vi "WLC for FA-50%GC_YCC.vi"() -> ()   [LabVIEW 2014]
uses:
  <vilib>/Utility/file.llb/Read From Spreadsheet File (DBL).vi
  <vilib>/gmath/NumericalOptimization/Nonlinear Curve Fit LM formula string.vi
  <vilib>/Utility/file.llb/Write To Spreadsheet File (DBL).vi
  <vilib>/gmath/NI_Gmath.lvlib
panel:
  out "reduced dsDNA (bp)":dbl=1002.0
  out "ssDNA generated (nt)":dbl
  out "Force Array  for activated best fit (pN)":dbl[](array[numeric])
  out "Extension array for activated best fit (nm)":dbl[](array[numeric])
  out "Force Array  for unactivated best fit (pN)":dbl[](array[numeric])
  out "Extension array for unactivated best fit (nm)":dbl[](array[numeric])
  in  "file path for activated  (dialog if empty) 2":path=path "D:/YCC/20190501/FA-2-S-great/221718-F+U-4500.00-3.00 um s^-1-L-9.37 nm avg step-FA-1-2-raw-U-ForecExtension Only.txt"
  out "Force for activated":dbl[](array[numeric])
  out "Extension for activated":dbl[](array[numeric])
  out "Cut-Ex for activated":dbl[](array[numeric])
  out "Cut-Force for activated":dbl[](array[numeric])
  in  "stop 2":bool
  in  "Save?":bool
  in  "stop":bool
  in  "file path for unactivated  (dialog if empty)":path=path "D:/YCC/20190501/FA-2-S-great/221718-F+U-4500.00-3.00 um s^-1-L-9.37 nm avg step-FA-1-2-raw-U-ForecExtension Only.txt"
  out "Cut-Force for unactivated":dbl[](array[numeric])
  out "Cut-Ex for unactivated":dbl[](array[numeric])
  in  "Tab Control":T1(tab)
  out "F-E curve":cluster{dbl[], dbl[]}(graph)
  out "XY Graph 6":cluster{"best nonlinear fit":dbl[], dbl[]}[](graph)
  out "best fit parameters":dbl[](array[numeric])
  in  "upper bound force (pN)":dbl=45.0
  in  "upper bound extension (nm)":dbl=2000.0
  in  "lower bound force (pN)":dbl=6.0
  in  "lower bound extension (nm)":dbl=400.0
  out "best fit Ex":dbl[](array[numeric])
  out "# of ssDNA nt for unactivated":dbl
  out "dsDNA bp for unactivated(nm)":dbl
  out "XY Graph 7":cluster{"best nonlinear fit":dbl[], dbl[]}[](graph)
  out "best fit Ex for activated":dbl[](array[numeric])
  out "best fit parameters 2":dbl[](array[numeric])
  in  "lower bound extension (nm)  2":dbl=400.0
  in  "upper bound extension (nm) 2":dbl=2000.0
  in  "upper bound force (pN)  2":dbl=46.0
  in  "lower bound force (pN) 2":dbl=15.0
  out "# of ssDNA nt for activated":dbl
  out "dsDNA bp for activated":dbl
  out "F-E curve 2":T2(graph)
  out "Extension for unactivated":dbl[](array[numeric])
  out "Force for unactivated":dbl[](array[numeric])
  # "5180 bp =\n1679+2411=4188 bp dsDNA=\n1002 ssDNA after activated\n\n0.338 nm/bp\n0.56 nm/nt"
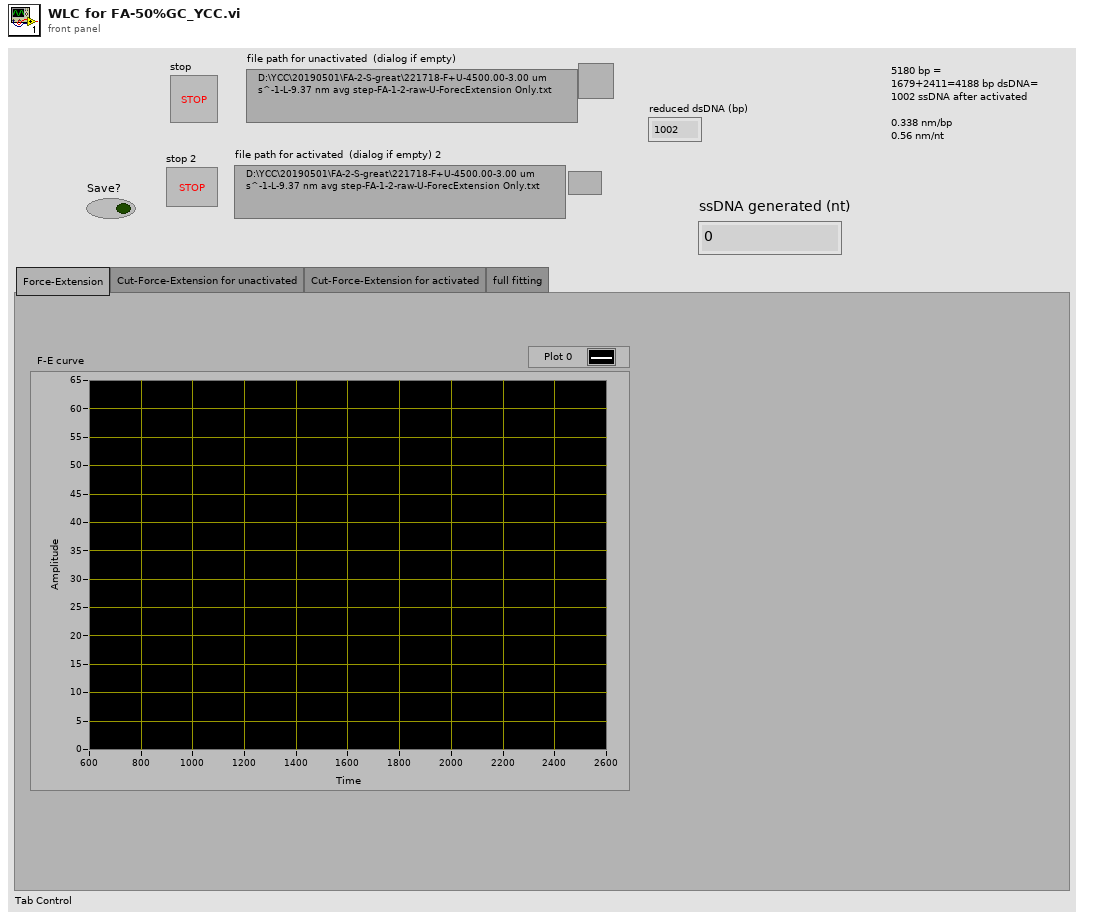
[diagram p1: front panel]
types:
  T1 = enum32{"Force-Extension", "Cut-Force-Extension for unactivated", "Cut-Force-Extension for activated", "full fitting"}
  T2 = cluster{"Extension for unactivated":dbl[], "Force for unactivated":dbl[]}[]
  T3 = cluster{"model":string, "Parameters":string[], "x":string}
  T4 = cluster{"Extension array (nm)":dbl[], "Force Array (pN)":dbl[]}
  T5 = cluster{"Extension for activated":dbl[], "Force for activated":dbl[]}
  T6 = cluster{"Extension for unactivated":dbl[], "Force for unactivated":dbl[]}
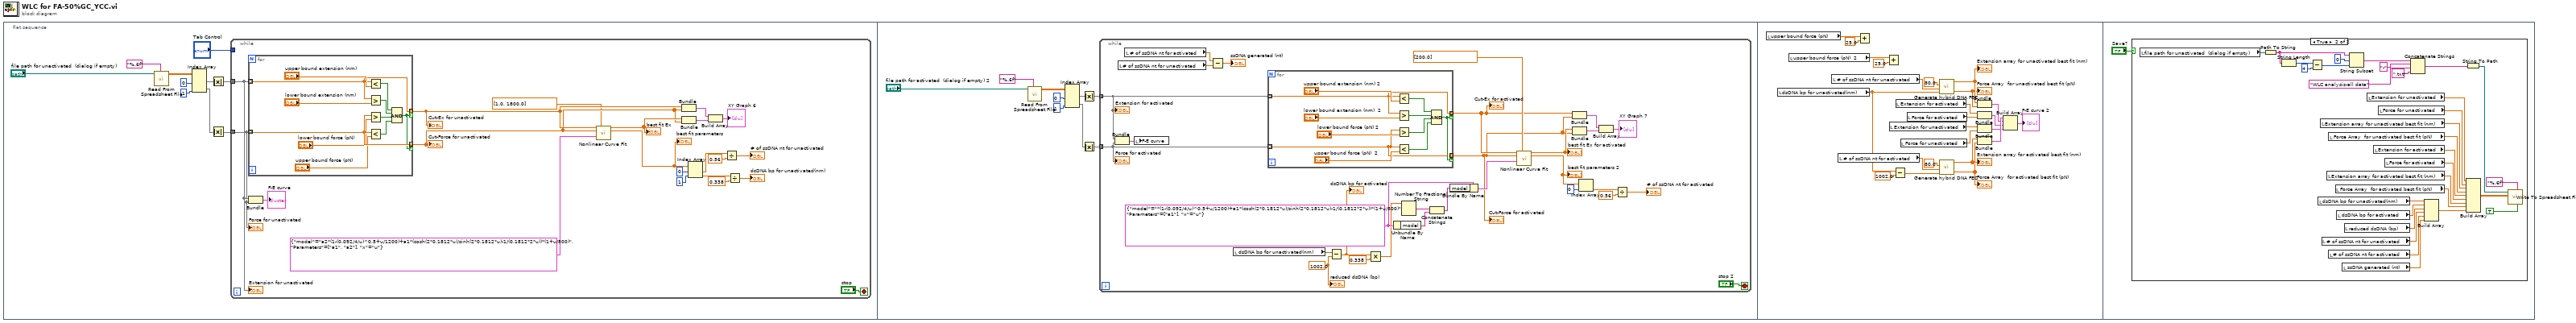
[diagram p0: block diagram]
diagram:
  n1 = flat-sequence {
    frame #0 {
      n2 = call-poly <vilib>:"Read From Spreadsheet File.vi"("format (%.3f)"="%.6f", "file path (dialog if empty)"="file path for unactivated  (dialog if empty)") -> ("all rows"=w1:dbl[][])  [unwired: 5 in, 4 out]
      n3 = Index Array(array=w1, index (col) #1=0 ("disabled index (col)"), index (col) #2=1 ("index (col)")) -> (element #1=w7:dbl[], element #2=w8:dbl[])  [unwired: 2 in]
      n4 = Absolute Value(x=w7) -> (abs(x)=w10:dbl[])
      n5 = Absolute Value(x=w8) -> (abs(x)=w9:dbl[])
      n6 = while {
        tunnel: w10 -> [w23]
        tunnel: w9 -> [w22]
        tunnel: "Tab Control" -> [_]
        stop <- "stop" stop-if-true
        n7 = for {
          tunnel: w22 -> [w42] mode=indexing
          tunnel: [w42] -> w28 mode=indexing if=w40
          tunnel: w23 -> [w35] mode=indexing
          tunnel: [w35] -> w31 mode=indexing if=w40
          n8 = Less?(x=w35, y="upper bound extension (nm)") -> (x < y?=w41:bool)
          n9 = Greater?(x=w35, y="lower bound extension (nm)") -> (0:w34:bool)
          n10 = Greater?(x=w42, y="lower bound force (pN)") -> (0:w33:bool)
          n11 = Less?(x=w42, y="upper bound force (pN)") -> (x < y?=w32:bool)
          n12 = Compound Arithmetic op=AND(w41, w34, w33, w32) -> (w40:bool)
        }
        "Cut-Ex for unactivated" <- w31
        "Cut-Force for unactivated" <- w28
        n13 = Bundle(w23, w22) -> (→"F-E curve":cluster{dbl[], dbl[]})  [unwired: 1 in]
        n14 = call-poly <vilib>:"Nonlinear Curve Fit.vi"("Y"=w31, "initial parameters"=dbl[] [1.0, 1800.0], "X"=w28, "model description"=T3 {"model"="a2*(1-(0.092/4/u)^0.5+u/1200)+a1*(cosh(2*0.1812*u)/sinh(2*0.1812*u)-1/(0.1812*2*u))*(1+u/800)", "Parameters"=["a1", "a2"], "x"="u"}) -> ("best nonlinear fit"=w29:dbl[], "best fit parameters"=w20:dbl[])  [unwired: 3 in, 7 out]
        "best fit parameters" <- w20
        "best fit Ex" <- w29
        n15 = Bundle(w31, w28) -> (w26:cluster{dbl[], dbl[]})  [unwired: 1 in]
        n16 = Bundle("best nonlinear fit"=w29, w28) -> (w25:cluster{"best nonlinear fit":dbl[], dbl[]})  [unwired: 1 in]
        n17 = Index Array(array=w20, index #1=0 ("index"), index #2=1 ("index")) -> (element #1=w18:dbl, element #2=w12:dbl)
        n18 = Build Array(w26, w25) -> (→"XY Graph 6":cluster{"best nonlinear fit":dbl[], dbl[]}[])
        n19 = Divide(x=w18, y=0.56) -> (x/y=→"# of ssDNA nt for unactivated":dbl)
        n20 = Divide(x=w12, y=0.338) -> (x/y=→"dsDNA bp for unactivated(nm)":dbl)
        "Force for unactivated" <- w22
        "Extension for unactivated" <- w23
      }
    }
    frame #1 {
      n21 = call-poly <vilib>:"Read From Spreadsheet File.vi"("format (%.3f)"="%.6f", "file path (dialog if empty)"="file path for activated  (dialog if empty) 2") -> ("all rows"=w45:dbl[][])  [unwired: 5 in, 4 out]
      n22 = Index Array(array=w45, index (col) #1=0 ("disabled index (col)"), index (col) #2=1 ("index (col)")) -> (element #1=w50:dbl[], element #2=w51:dbl[])  [unwired: 2 in]
      n23 = Absolute Value(x=w50) -> (abs(x)=w44:dbl[])
      n24 = Absolute Value(x=w51) -> (abs(x)=w43:dbl[])
      n25 = while {
        tunnel: w44 -> [w58]
        tunnel: w43 -> [w57]
        stop <- "stop 2" stop-if-true
        w52 = 1002.0 ("y")
        w68 = T3 {"model"="*(1-(0.092/4/u)^0.5+u/1200)+a1*(cosh(2*0.1812*u)/sinh(2*0.1812*u)-1/(0.1812*2*u))*(1+u/800)", "Parameters"=["a1"], "x"="u"} ("model description")
        n26 = Bundle(w58, w57) -> (w56:cluster{dbl[], dbl[]})  [unwired: 1 in]
        n27 = local read "# of ssDNA nt for unactivated"() -> (w54:dbl)
        n28 = local read "# of ssDNA nt for activated"() -> (w53:dbl)
        n29 = local write "F-E curve"(w56) -> ()
        n30 = Subtract(x=w53, y=w54) -> (x-y=→"ssDNA generated (nt)":dbl)
        n31 = local read "dsDNA bp for unactivated(nm)"() -> (w62:dbl)
        n32 = for {
          tunnel: [w81] -> w63 mode=indexing if=w90
          tunnel: [w82] -> w64 mode=indexing if=w90
          tunnel: w58 -> [w82] mode=indexing
          tunnel: w57 -> [w81] mode=indexing
          n33 = Less?(x=w82, y="upper bound extension (nm) 2") -> (x < y?=w91:bool)
          n34 = Greater?(x=w82, y="lower bound extension (nm)  2") -> (0:w85:bool)
          n35 = Greater?(x=w81, y="lower bound force (pN) 2") -> (0:w84:bool)
          n36 = Less?(x=w81, y="upper bound force (pN)  2") -> (x < y?=w83:bool)
          n37 = Compound Arithmetic op=AND(w91, w85, w84, w83) -> (w90:bool)
        }
        "Cut-Ex for activated" <- w64
        "Cut-Force for activated" <- w63
        n38 = Subtract(x=w62, y=w52) -> (x-y=w61:dbl)
        "dsDNA bp for activated" <- w61
        n39 = Multiply(x=w61, y=0.338) -> (x*y=w59:dbl)
        n40 = Unbundle By Name(w68) -> ("model"=w70:string)
        n41 = Number To Fractional String(number=w59) -> (F-format string=w69:string)  [unwired: 3 in]
        n42 = Concatenate Strings(w69, w70) -> (w67:string)
        n43 = Bundle By Name(cluster=w68, "model"=w67) -> (w80:T3)
        n44 = call-poly <vilib>:"Nonlinear Curve Fit.vi"("Y"=w64, "initial parameters"=dbl[] [200.0], "X"=w63, "model description"=w80) -> ("best nonlinear fit"=w79:dbl[], "best fit parameters"=w76:dbl[])  [unwired: 3 in, 7 out]
        "best fit parameters 2" <- w76
        "best fit Ex for activated" <- w79
        n45 = Bundle(w64, w63) -> (w66:cluster{dbl[], dbl[]})  [unwired: 1 in]
        n46 = Bundle("best nonlinear fit"=w79, w63) -> (w78:cluster{"best nonlinear fit":dbl[], dbl[]})  [unwired: 1 in]
        n47 = Index Array(array=w76, index=0) -> (element=w74:dbl)
        n48 = Build Array(w66, w78) -> (→"XY Graph 7":cluster{"best nonlinear fit":dbl[], dbl[]}[])
        n49 = Divide(x=w74, y=0.56) -> (x/y=→"# of ssDNA nt for activated":dbl)
        "Force for activated" <- w57
        "Extension for activated" <- w58
        "reduced dsDNA (bp)" <- w52
      }
    }
    frame #2 {
      n50 = local read "upper bound force (pN)"() -> (w94:dbl)
      n51 = local read "dsDNA bp for unactivated(nm)"() -> (w111:dbl)
      n52 = local read "upper bound force (pN)  2"() -> (w97:dbl)
      n53 = local read "# of ssDNA nt for unactivated"() -> (w115:dbl)
      n54 = local read "# of ssDNA nt for activated"() -> (w114:dbl)
      n55 = Add(x=w94, y=25.0) -> ()  [unwired: 1 out]
      n56 = Add(x=w97, y=25.0) -> ()  [unwired: 1 out]
      n57 = local read "Extension for unactivated"() -> (w106:dbl[])
      n58 = Subtract(x=w111, y=1002.0) -> (x-y=w112:dbl)
      n59 = local read "Extension for activated"() -> (w104:dbl[])
      n60 = local read "Force for unactivated"() -> (w105:dbl[])
      n61 = local read "Force for activated"() -> (w103:dbl[])
      n62 = call "Generate hybrid DNA FEC.vi"("End Force (pN)"=80.0, "ssDNA Length (nt)"=w115, "dsDNA Length (bp)"=w111) -> ("Extension array (nm)"=w110:dbl[], "Force Array (pN)"=w109:dbl[])  [unwired: 2 in, 2 out]
      "Extension array for unactivated best fit (nm)" <- w110
      "Force Array  for unactivated best fit (pN)" <- w109
      n63 = call "Generate hybrid DNA FEC.vi"("End Force (pN)"=80.0, "ssDNA Length (nt)"=w114, "dsDNA Length (bp)"=w112) -> ("Extension array (nm)"=w108:dbl[], "Force Array (pN)"=w107:dbl[])  [unwired: 2 in, 2 out]
      "Extension array for activated best fit (nm)" <- w108
      "Force Array  for activated best fit (pN)" <- w107
      n64 = Bundle("Extension array (nm)"=w110, "Force Array (pN)"=w109) -> (w101:T4)  [unwired: 1 in]
      n65 = Bundle("Extension for activated"=w104, "Force for activated"=w103) -> (w100:T5)  [unwired: 1 in]
      n66 = Bundle("Extension for unactivated"=w106, "Force for unactivated"=w105) -> (w99:T6)  [unwired: 1 in]
      n67 = Bundle("Extension array (nm)"=w108, "Force Array (pN)"=w107) -> (w102:T4)  [unwired: 1 in]
      n68 = Build Array(w102, w101, w100, w99) -> (→"F-E curve 2":T2)
    }
    frame #3 {
      n69 = case shown="True" "Save?" {
        frame False {
        }
        frame True {
          n70 = local read "file path for unactivated  (dialog if empty)"() -> (w139:path)
          n71 = Path To String(path=w139) -> (string=w134:string)
          n72 = String Length(string=w134) -> (length=w135:i32)
          n73 = Subtract(x=w135, y=4) -> (x-y=w138:i32)
          n74 = local read "dsDNA bp for unactivated(nm)"() -> (w119:dbl)
          n75 = local read "Extension array for unactivated best fit (nm)"() -> (w130:dbl[])
          n76 = local read "# of ssDNA nt for unactivated"() -> (w124:dbl)
          n77 = local read "Extension array for activated best fit (nm)"() -> (w126:dbl[])
          n78 = local read "# of ssDNA nt for activated"() -> (w123:dbl)
          n79 = local read "Force Array  for unactivated best fit (pN)"() -> (w129:dbl[])
          n80 = local read "Force Array  for activated best fit (pN)"() -> (w125:dbl[])
          n81 = local read "dsDNA bp for activated"() -> (w118:dbl)
          n82 = local read "ssDNA generated (nt)"() -> (w120:dbl)
          n83 = local read "reduced dsDNA (bp)"() -> (w117:dbl)
          n84 = String Subset(string=w134, offset (0)=0, length (rest)=w138) -> (substring=w143:string)
          n85 = local read "Extension for unactivated"() -> (w132:dbl[])
          n86 = local read "Extension for activated"() -> (w128:dbl[])
          n87 = local read "Force for unactivated"() -> (w131:dbl[])
          n88 = local read "Force for activated"() -> (w127:dbl[])
          n89 = Concatenate Strings(w143, "-" ("string"), "WLC analysis-all data" ("string"), ".txt" ("string")) -> (w140:string)
          n90 = Build Array(w119, w118, w117, w124, w123, w120) -> (w122:dbl[])
          n91 = String To Path(string=w140) -> (path=w133:path)
          n92 = Build Array(w132, w131, w130, w129, w128, w127, w126, w125, w122) -> (w121:dbl[][])
          n93 = call-poly <vilib>:"Write To Spreadsheet File.vi"("transpose? (no:F)"=TRUE, "format (%.3f)"="%.6f", "2D data"=w121, "file path (dialog if empty)"=w133) -> ()  [unwired: 4 in, 1 out]
        }
      }
    }
  }
